vi "Theta 3.vi"(5 "XYZ_6012":dbl[](array[numeric])=[0.0, 0.0, 0.0], 7 "XYZbar_4":dbl[](array[numeric])=[0.0, 0.0, 0.0], 11 "6R Type 2 Serial Arm Class in":refnum<class "NI_Robotics_6R Type 2 Serial Arm Class.lvclass">) -> (1 "Valid":bool, 2 "theta_3":dbl, 3 "6R Type 2 Serial Arm Class out":refnum<class "NI_Robotics_6R Type 2 Serial Arm Class.lvclass">)   [LabVIEW 2017, in "NI_Robotics_6R Type 2 Serial Arm Class.lvclass"]
uses:
  <vilib>/robotics/Kinematics/Analytical/6R/Type 2/NI_Robotics_6R Type 2 Serial Arm Class.lvclass
  <vilib>/Analysis/7linalg.llb/Solve Linear Equations (single right hand).vi
  <vilib>/Analysis/baseanly.llb/Solve Linear Equations By Cholesky.vi
  <vilib>/Analysis/baseanly.llb/Real Matrix to Compact Array.vi
  <vilib>/Analysis/baseanly.llb/Real Compact Tri-Matrix Linear Eqs.vi
  <vilib>/Analysis/7linalg.llb/Solve Linear Eqs (General).vi
  <vilib>/Analysis/7linalg.llb/Solve Linear Eqs (Gen, single right hand).vi
  <vilib>/Analysis/NI_AALPro.lvlib
panel:
  out "Solution Vector":dbl[](array[numeric]) format="%.5f"
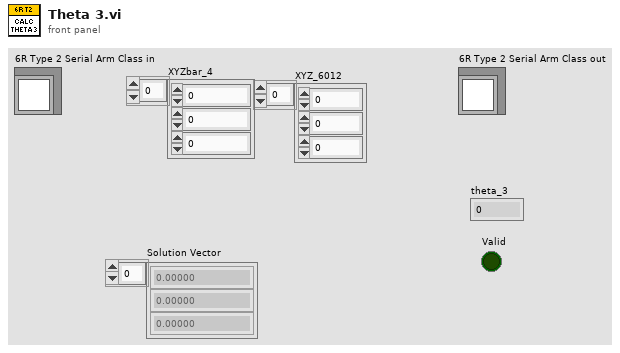
[diagram p1: front panel]
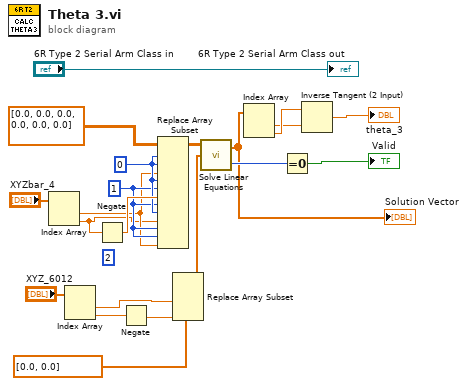
[diagram p0: block diagram]
diagram:
  (unwired) 2 ("disabled index (col)")
  w7 = 1 ("disabled index (col)")
  w8 = 0 ("index (row)")
  n1 = Index Array(array="XYZbar_4") -> (element #1=w6:dbl, element #2=w5:dbl)  [unwired: 2 in]
  n2 = Index Array(array="XYZ_6012") -> (element #1=w2:dbl, element #2=w20:dbl)  [unwired: 2 in]
  n3 = Negate(x=w5) -> (-x=w9:dbl)
  n4 = Negate(x=w20) -> (-x=w3:dbl)
  n5 = Replace Array Subset(array=dbl[][] [[0.0, 0.0, 0.0], [0.0, 0.0, 0.0]], new element #1=w6, index (row) #1=w8, index (col) #1=w8, new element #2=w9, index (row) #2=w8, index (col) #2=w7, new element #3=w5, index (row) #3=w7, index (col) #3=w8, new element #4=w6, index (row) #4=w7, index (col) #4=w7) -> (w16:dbl[][])
  n6 = Replace Array Subset(array=dbl[] [0.0, 0.0], new element #1=w2, new element #2=w3) -> (w1:dbl[])  [unwired: 2 in]
  n7 = call-poly <vilib>:"Solve Linear Equations.vi"("Known Vector"=w1, "Input Matrix"=w16) -> ("error"=w18:i32, "Solution Vector"=w17:dbl[])  [unwired: 1 in]
  "Solution Vector" <- w17
  n8 = Index Array(array=w17) -> (element #1=w10:dbl, element #2=w11:dbl)  [unwired: 2 in]
  n9 = Equal To 0?(x=w18) -> (x = 0?=→"Valid":bool)
  n10 = Inverse Tangent (2 Input)(1:w10, 2:w11) -> (0:→"theta_3":dbl)
  "6R Type 2 Serial Arm Class out" <- "6R Type 2 Serial Arm Class in"
